vi "Pockels Cal-Source-Wizard states array.vi"() -> (3 "States sequence":T1[](array[typedef]))   [LabVIEW 2020]
uses:
  Typedefs/Pockels cal wizard states.ctl
  Globals/gl_Calibration globals.vi
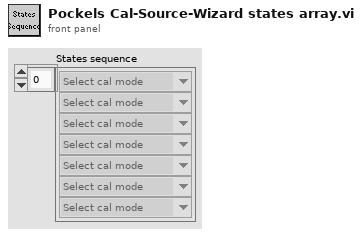
[diagram p1: front panel]
types:
  T1 = typedef "Pockels cal wizard states.ctl" = enum16{"Select cal mode", "Show instructions 1", "Select channel", "Show instructions 2", "Show instructions 3", "Confirm start", "Start calibration"}
  T2 = typedef "Cal mode.ctl" = enum16{"Automatic", "Interactive"}
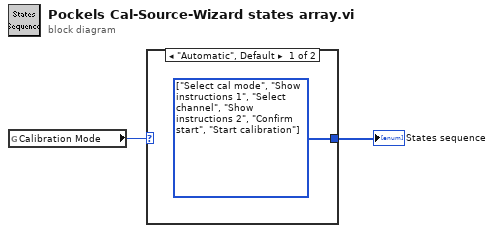
[diagram p0: block diagram]
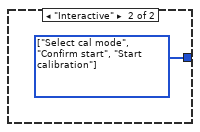
[diagram p2: hidden frame]
diagram:
  n1 = global read "gl_Calibration globals.vi" "Calibration Mode"() -> (w1:T2)
  n2 = case shown="\"Automatic\", Default" w1 {
    tunnel: [w3 w4] -> w2
    frame "Automatic", Default {
      w3 = T1[] [enum."Select cal mode", enum."Show instructions 1", enum."Select channel", enum."Show instructions 2", enum."Confirm start", enum."Start calibration"] items=["Select cal mode", "Show instructions 1", "Select channel", "Show instructions 2", "Show instructions 3", "Confirm start", "Start calibration"]
    }
    frame "Interactive" {
      w4 = T1[] [enum."Select cal mode", enum."Confirm start", enum."Start calibration"] items=["Select cal mode", "Show instructions 1", "Select channel", "Show instructions 2", "Show instructions 3", "Confirm start", "Start calibration"]
    }
  }
  "States sequence" <- w2
